vi "Simple TCP - Server.vi"() -> ()   [LabVIEW 2021]
doc: "Demonstrates how to set up a basic TCP connection, send data to the specified port once a connection has been established, and terminate the connection once the data has been sent. This VI is designed to stop if the TCP connection is terminated. The data sent in this example is an array of random numbers."
panel:
  in  "?":path
  in  "Client Closed":string="The client VI closed the connection."
  in  "Stop":bool
  # "choose file send to client"
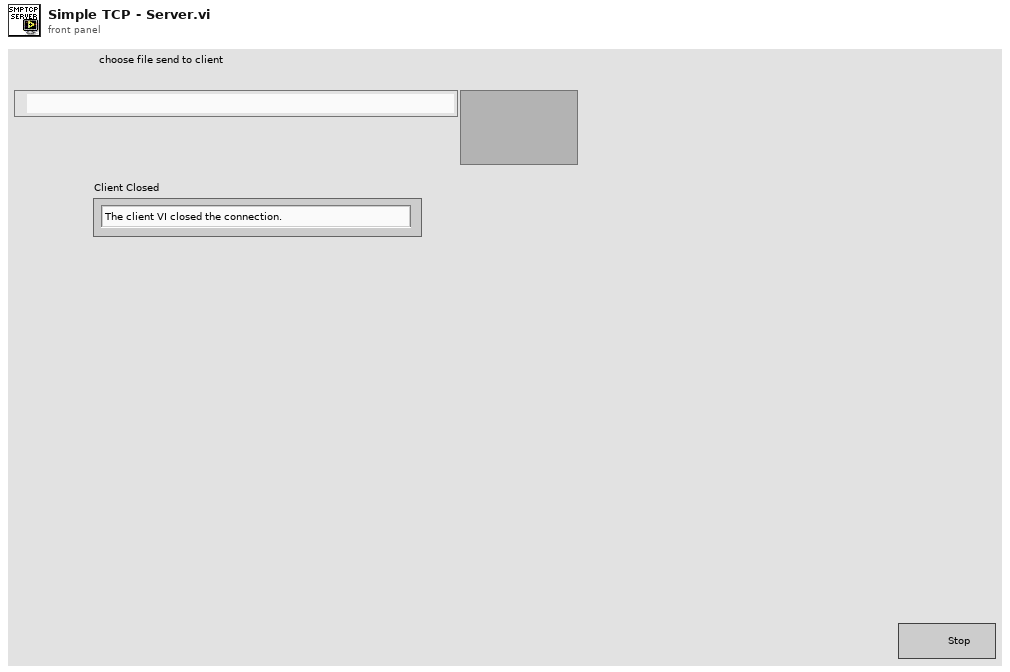
[diagram p1: front panel]
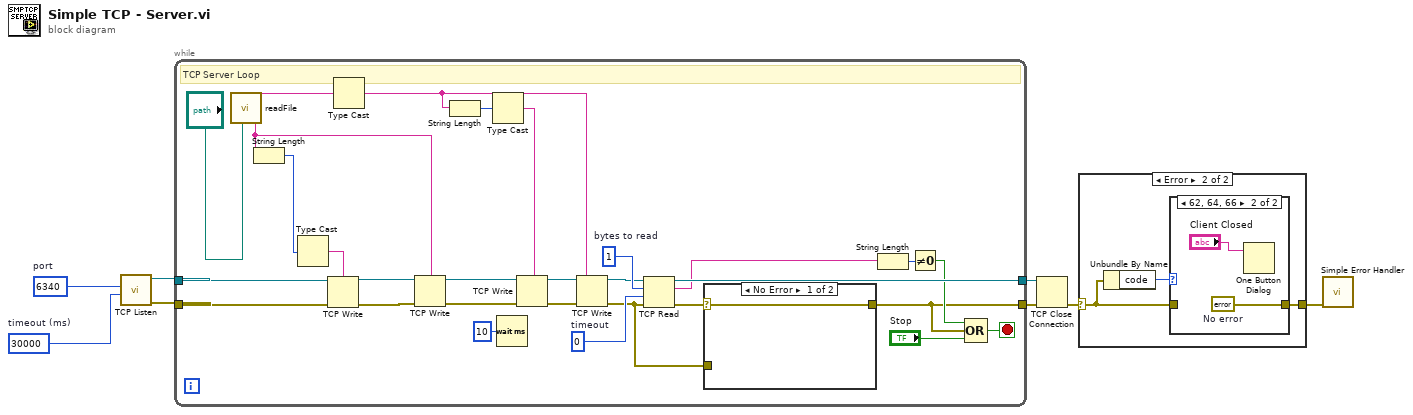
[diagram p0: block diagram]
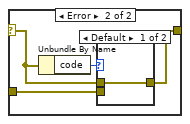
[diagram p4: hidden frame]
diagram:
  w1 = u16 6340  # port
  w2 = 30000  # timeout (ms)
  n1 = call <vilib>:"TCP Listen.vi"("timeout ms (wait forever: -1)"=w2, "port"=w1) -> ("error out"=w3:errorcluster, "connection ID"=w4:refnum<k5>)  [unwired: 5 in, 3 out]
  n2 = while {
    tunnel: [w21] -> w7
    tunnel: [w27] -> w8
    tunnel: w4 -> [w16]
    tunnel: w3 -> [w17]
    stop <- w31 stop-if-true
    w26 = 0  # timeout
    w29 = 1  # bytes to read
    # "TCP Server Loop"
    n3 = call "readFile.vi"("name or relative path"="?") -> ("fileName"=w9:string, "dataOut"=w19:string)  [unwired: 9 in]
    n4 = String Length(string=w9) -> (length=w11:i32)
    n5 = Type Cast(x=w11) -> (*(type *) &x=w10:string)  [unwired: 1 in]
    n6 = TCP Write(connection ID=w16, data in=w10, error in (no error)=w17) -> (connection ID out=w15:refnum<k5>, error out=w13:errorcluster)  [unwired: 1 in, 1 out]
    n7 = Type Cast(x=w19) -> (*(type *) &x=w33:string)  [unwired: 1 out]
    n8 = TCP Write(connection ID=w15, data in=w9, error in (no error)=w13) -> (connection ID out=w14:refnum<k5>, error out=w12:errorcluster)  [unwired: 1 in, 1 out]
    n9 = String Length(string=w33) -> (length=w35:i32)
    n10 = Type Cast(x=w35) -> (*(type *) &x=w34:string)  [unwired: 1 out]
    n11 = Wait (ms)(milliseconds to wait=u32 10) -> ()  [unwired: 1 out]
    n12 = TCP Write(connection ID=w14, data in=w34, error in (no error)=w12) -> (connection ID out=w37:refnum<k5>, error out=w36:errorcluster)  [unwired: 2 out]
    n13 = TCP Write(connection ID=w37, data in=w33, error in (no error)=w36) -> (connection ID out=w28:refnum<k5>, error out=w20:errorcluster)  [unwired: 2 out]
    n14 = TCP Read(connection ID=w28, bytes to read=w29, error in (no error)=w20, 9:w26) -> (connection ID out=w27:refnum<k5>, data out=w24:string, error out=w22:errorcluster)  [unwired: 1 out]
    n15 = case shown="No Error" w22 {
      selector: w22 -> [w38 w41]
      tunnel: [w38 w39] -> w21
      tunnel: w20 -> [_ w40]
      frame No Error {
      }
      frame Error {
        n16 = Unbundle By Name(w41) -> ("code"=w42:i32)
        n17 = case shown="Default" w42 {
          tunnel: w41 -> [w43 _]
          tunnel: w40 -> [_ w44]
          tunnel: [w43 w44] -> w39
          frame Default {
          }
          frame 56 {
          }
        }
      }
    }
    n18 = String Length(string=w24) -> (length=w25:i32)
    n19 = Not Equal To 0?(x=w25) -> (x != 0?=w23:bool)
    n20 = Compound Arithmetic op=OR(w23, w21, "Stop") -> (w31:bool)
  }
  n21 = TCP Close Connection(connection ID=w8, error in (no error)=w7) -> (error out=w6:errorcluster)  [unwired: 2 out]
  n22 = case shown="Error" w6 {
    selector: w6 -> [w45 w47]
    tunnel: [w45 w46] -> w5
    frame No Error {
    }
    frame Error {
      n23 = Unbundle By Name(w47) -> ("code"=w48:i32)
      n24 = case shown="62, 64, 66" w48 {
        tunnel: w47 -> [w49 _]
        tunnel: [w49 w51] -> w46
        frame Default {
        }
        frame 62, 64, 66 {
          w51 = errorcluster {"status"=FALSE, "code"=0, "source"=""}  # No error
          n25 = One Button Dialog(message="Client Closed") -> ()  [unwired: 1 in, 1 out]
        }
      }
    }
  }
  n26 = call <vilib>:"Simple Error Handler.vi"("error in (no error)"=w5) -> ()  [unwired: 1 in, 8 out]
